vi "nanocal -- nuclear schottky fit V8.vi"() -> ()   [LabVIEW 2021] (continued)
τC\" -> 0.000802475621   ,  \"κ0\" -> 0.000000000773   ,  \"mm1\" -> 0.000163026258   ,  \"mm2\" -> 0.019497997616   ,  \"mm3\" -> 0.165534595934   ,  \"T\" -> 0.190000000000   ,  \"B\" -> 10.000000000000   ,  \"θ\" -> 0.000000000000   ,  \"Reoff\" -> -55142857.142857134400   ,  \"Imoff\" -> 0.000000000000   ,  \"στ1\" -> 0.000058307175   ,  \"στS\" -> 0.000031998048   ,  \"στN\" -> 0.000036682192   ,  \"τ11 \" -> 0.000000000000   ,  \"τ12\" -> 0.000000000000   ,  \"τ22\" -> 0.000000000000   ,  \"τN1\" -> 0.000000000000   ,  \"τN2\" -> 0.000000000000   ,  \"σηlogτ1 \" -> 0.000000000000   ,  \"σηlogτS\" -> 0.000000000000   ,  \"σηlogτN\" -> 0.000000000000   ,  \"σlogτ1\" -> 0.000000000000   ,  \"σlogτS\" -> 0.000000000000   ,  \"σlogτN\" -> 0.000000000000   ,  \"σητ1\" -> 0.000000000000   ,  \"σητS \" -> 0.000000000000   ,  \"σητN\" -> 0.000000000000    |>   , \n\"IDS0424_220526_RAW_cal__sam_\" ->   <|    \"ζ\" -> 0.143096873941   ,  \"τ1\" -> 0.119527741552   ,  \"τS\" -> 0.213771204505   ,  \"τN\" -> 0.133065206622   ,  \"τC\" -> 0.001041786526   ,  \"κ0\" -> 0.000000000890   ,  \"mm1\" -> 0.000129929317   ,  \"mm2\" -> 0.064852834373   ,  \"mm3\" -> 0.452054381716   ,  \"T\" -> 0.190000000000   ,  \"B\" -> 10.000000000000   ,  \"θ\" -> 0.000000000000   ,  \"Reoff\" -> -41461224.489795915800   ,  \"Imoff\" -> 0.000000000000   ,  \"στ1\" -> 0.142328196867   ,  \"στS\" -> 0.153709890516   ,  \"στN\" -> 0.034979737706   ,  \"τ11 \" -> 0.000000000000   ,  \"τ12\" -> 0.000000000000   ,  \"τ22\" -> 0.000000000000   ,  \"τN1\" -> 0.000000000000   ,  \"τN2\" -> 0.000000000000   ,  \"σηlogτ1 \" -> 0.000000000000   ,  \"σηlogτS\" -> 0.000000000000   ,  \"σηlogτN\" -> 0.000000000000   ,  \"σlogτ1\" -> 0.000000000000   ,  \"σlogτS\" -> 0.000000000000   ,  \"σlogτN\" -> 0.000000000000   ,  \"σητ1\" -> 0.000000000000   ,  \"σητS \" -> 0.000000000000   ,  \"σητN\" -> 0.000000000000    |>   , \n\"IDS0425_220526_RAW_cal__ref_\" ->   <|    \"ζ\" -> 0.159335076752   ,  \"τ1\" -> 0.031885685275   ,  \"τS\" -> 0.047996731633   ,  \"τN\" -> 0.019207310502   ,  \"τC\" -> 0.000887935907   ,  \"κ0\" -> 0.000000001118   ,  \"mm1\" -> 0.000120371950   ,  \"mm2\" -> 0.019822778110   ,  \"mm3\" -> 0.090742474469   ,  \"T\" -> 0.250000000000   ,  \"B\" -> 10.000000000000   ,  \"θ\" -> 0.000000000000   ,  \"Reoff\" -> -27579558.011049721400   ,  \"Imoff\" -> 0.000000000000   ,  \"στ1\" -> 0.000105033309   ,  \"στS\" -> 0.000027614157   ,  \"στN\" -> 0.000060474658   ,  \"τ11 \" -> 0.000000000000   ,  \"τ12\" -> 0.000000000000   ,  \"τ22\" -> 0.000000000000   ,  \"τN1\" -> 0.000000000000   ,  \"τN2\" -> 0.000000000000   ,  \"σηlogτ1 \" -> 0.000000000000   ,  \"σηlogτS\" -> 0.000000000000   ,  \"σηlogτN\" -> 0.000000000000   ,  \"σlogτ1\" -> 0.000000000000   ,  \"σlogτS\" -> 0.000000000000   ,  \"σlogτN\" -> 0.000000000000   ,  \"σητ1\" -> 0.000000000000   ,  \"σητS \" -> 0.000000000000   ,  \"σητN\" -> 0.000000000000    |>   , \n\"IDS0425_220526_RAW_cal__sam_\" ->   <|    \"ζ\" -> 0.080613368975   ,  \"τ1\" -> 0.039981630615   ,  \"τS\" -> 0.067451052819   ,  \"τN\" -> 0.024952731947   ,  \"τC\" -> 0.001301901326   ,  \"κ0\" -> 0.000000001270   ,  \"mm1\" -> 0.000095538727   ,  \"mm2\" -> 0.025680137218   ,  \"mm3\" -> 0.115360621158   ,  \"T\" -> 0.250000000000   ,  \"B\" -> 10.000000000000   ,  \"θ\" -> 0.000000000000   ,  \"Reoff\" -> -15077551.020408168400   ,  \"Imoff\" -> 0.000000000000   ,  \"στ1\" -> 0.017921325903   ,  \"στS\" -> 0.008554959302   ,  \"στN\" -> 0.012696106226   ,  \"τ11 \" -> 0.000000000000   ,  \"τ12\" -> 0.000000000000   ,  \"τ22\" -> 0.000000000000   ,  \"τN1\" -> 0.000000000000   ,  \"τN2\" -> 0.000000000000   ,  \"σηlogτ1 \" -> 0.000000000000   ,  \"σηlogτS\" -> 0.000000000000   ,  \"σηlogτN\" -> 0.000000000000   ,  \"σlogτ1\" -> 0.000000000000   ,  \"σlogτS\" -> 0.000000000000   ,  \"σlogτN\" -> 0.000000000000   ,  \"σητ1\" -> 0.000000000000   ,  \"σητS \" -> 0.000000000000   ,  \"σητN\" -> 0.000000000000    |>   , \n\"IDS0426_220526_RAW_cal__ref_\" ->   <|    \"ζ\" -> 0.111460827005   ,  \"τ1\" -> 0.024224453348   ,  \"τS\" -> 0.042028783084   ,  \"τN\" -> 0.009416687783   ,  \"τC\" -> 0.001053496592   ,  \"κ0\" -> 0.000000001428   ,  \"mm1\" -> 0.000103540379   ,  \"mm2\" -> 0.017919606240   ,  \"mm3\" -> 0.064434428916   ,  \"T\" -> 0.300000000000   ,  \"B\" -> 10.000000000000   ,  \"θ\" -> 0.000000000000   ,  \"Reoff\" -> -13408163.265306122600   ,  \"Imoff\" -> 0.000000000000   ,  \"στ1\" -> 0.000203310758   ,  \"στS\" -> 0.000031022481   ,  \"στN\" -> 0.000119793909   ,  \"τ11 \" -> 0.000000000000   ,  \"τ12\" -> 0.000000000000   ,  \"τ22\" -> 0.000000000000   ,  \"τN1\" -> 0.000000000000   ,  \"τN2\" -> 0.000000000000   ,  \"σηlogτ1 \" -> 0.000000000000   ,  \"σηlogτS\" -> 0.000000000000   ,  \"σηlogτN\" -> 0.000000000000   ,  \"σlogτ1\" -> 0.000000000000   ,  \"σlogτS\" -> 0.000000000000   ,  \"σlogτN\" -> 0.000000000000   ,  \"σητ1\" -> 0.000000000000   ,  \"σητS \" -> 0.000000000000   ,  \"σητN\" -> 0.000000000000    |>   , \n\"IDS0426_220526_RAW_cal__sam_\" ->   <|    \"ζ\" -> 0.000000000000   ,  \"τ1\" -> 0.000000000000   ,  \"τS\" -> 0.000000000000   ,  \"τN\" -> 0.000000000000   ,  \"τC\" -> 0.000000000000   ,  \"κ0\" -> 0.000000000000   ,  \"mm1\" -> 0.000000000000   ,  \"mm2\" -> 0.000000000000   ,  \"mm3\" -> 0.000000000000   ,  \"T\" -> 0.300000000000   ,  \"B\" -> 10.000000000000   ,  \"θ\" -> 0.000000000000   ,  \"Reoff\" -> 0.000000000000   ,  \"Imoff\" -> 0.000000000000   ,  \"στ1\" -> 0.000000000000   ,  \"στS\" -> 0.000000000000   ,  \"στN\" -> 0.000000000000   ,  \"τ11 \" -> 0.000000000000   ,  \"τ12\" -> 0.000000000000   ,  \"τ22\" -> 0.000000000000   ,  \"τN1\" -> 0.000000000000   ,  \"τN2\" -> 0.000000000000   ,  \"σηlogτ1 \" -> 0.000000000000   ,  \"σηlogτS\" -> 0.000000000000   ,  \"σηlogτN\" -> 0.000000000000   ,  \"σlogτ1\" -> 0.000000000000   ,  \"σlogτS\" -> 0.000000000000   ,  \"σlogτN\" -> 0.000000000000   ,  \"σητ1\" -> 0.000000000000   ,  \"σητS \" -> 0.000000000000   ,  \"σητN\" -> 0.000000000000    |>   , \n\"IDS0427_220526_RAW_cal__ref_\" ->   <|    \"ζ\" -> 0.410372558234   ,  \"τ1\" -> 0.044042677076   ,  \"τS\" -> 0.102926494068   ,  \"τN\" -> 0.135379226142   ,  \"τC\" -> 0.000829804272   ,  \"κ0\" -> 0.000000000538   ,  \"mm1\" -> 0.000240462729   ,  \"mm2\" -> 0.017682403463   ,  \"mm3\" -> 0.363049463410   ,  \"T\" -> 0.150000000000   ,  \"B\" -> 10.000000000000   ,  \"θ\" -> 0.000000000000   ,  \"Reoff\" -> -106571428.571428567000   ,  \"Imoff\" -> 0.000000000000   ,  \"στ1\" -> 0.000056157157   ,  \"στS\" -> 0.000057678080   ,  \"στN\" -> 0.000041998406   ,  \"τ11 \" -> 0.000000000000   ,  \"τ12\" -> 0.000000000000   ,  \"τ22\" -> 0.000000000000   ,  \"τN1\" -> 0.000000000000   ,  \"τN2\" -> 0.000000000000   ,  \"σηlogτ1 \" -> 0.000000000000   ,  \"σηlogτS\" -> 0.000000000000   ,  \"σηlogτN\" -> 0.000000000000   ,  \"σlogτ1\" -> 0.000000000000   ,  \"σlogτS\" -> 0.000000000000   ,  \"σlogτN\" -> 0.000000000000   ,  \"σητ1\" -> 0.000000000000   ,  \"σητS \" -> 0.000000000000   ,  \"σητN\" -> 0.000000000000    |>   , \n\"IDS0427_220526_RAW_cal__sam_\" ->   <|    \"ζ\" -> 0.000000000000   ,  \"τ1\" -> 0.000000000000   ,  \"τS\" -> 0.000000000000   ,  \"τN\" -> 0.000000000000   ,  \"τC\" -> 0.000000000000   ,  \"κ0\" -> 0.000000000000   ,  \"mm1\" -> 0.000000000000   ,  \"mm2\" -> 0.000000000000   ,  \"mm3\" -> 0.000000000000   ,  \"T\" -> 0.150000000000   ,  \"B\" -> 10.000000000000   ,  \"θ\" -> 0.000000000000   ,  \"Reoff\" -> 0.000000000000   ,  \"Imoff\" -> 0.000000000000   ,  \"στ1\" -> 0.000000000000   ,  \"στS\" -> 0.000000000000   ,  \"στN\" -> 0.000000000000   ,  \"τ11 \" -> 0.000000000000   ,  \"τ12\" -> 0.000000000000   ,  \"τ22\" -> 0.000000000000   ,  \"τN1\" -> 0.000000000000   ,  \"τN2\" -> 0.000000000000   ,  \"σηlogτ1 \" -> 0.000000000000   ,  \"σηlogτS\" -> 0.000000000000   ,  \"σηlogτN\" -> 0.000000000000   ,  \"σlogτ1\" -> 0.000000000000   ,  \"σlogτS\" -> 0.000000000000   ,  \"σlogτN\" -> 0.000000000000   ,  \"σητ1\" -> 0.000000000000   ,  \"σητS \" -> 0.000000000000   ,  \"σητN\" -> 0.000000000000    |>   , \n\"IDS0428_220526_RAW_cal__ref_\" ->   <|    \"ζ\" -> 0.085761087931   ,  \"τ1\" -> 0.025055116447   ,  \"τS\" -> 0.039037181879   ,  \"τN\" -> 0.005587062279   ,  \"τC\" -> 0.001009401057   ,  \"κ0\" -> 0.000000001845   ,  \"mm1\" -> 0.000078014543   ,  \"mm2\" -> 0.019900208864   ,  \"mm3\" -> 0.054537561983   ,  \"T\" -> 0.360000000000   ,  \"B\" -> 10.000000000000   ,  \"θ\" -> 0.000000000000   ,  \"Reoff\" -> -10418232.044198893000   ,  \"Imoff\" -> 0.000000000000   ,  \"στ1\" -> 0.000347384848   ,  \"στS\" -> 0.000031989956   ,  \"στN\" -> 0.000188370043   ,  \"τ11 \" -> 0.000000000000   ,  \"τ12\" -> 0.000000000000   ,  \"τ22\" -> 0.000000000000   ,  \"τN1\" -> 0.000000000000   ,  \"τN2\" -> 0.000000000000   ,  \"σηlogτ1 \" -> 0.000000000000   ,  \"σηlogτS\" -> 0.000000000000   ,  \"σηlogτN\" -> 0.000000000000   ,  \"σlogτ1\" -> 0.000000000000   ,  \"σlogτS\" -> 0.000000000000   ,  \"σlogτN\" -> 0.000000000000   ,  \"σητ1\" -> 0.000000000000   ,  \"σητS \" -> 0.000000000000   ,  \"σητN\" -> 0.000000000000    |>   , \n\"IDS0428_220526_RAW_cal__sam_\" ->   <|    \"ζ\" -> 0.000000000000   ,  \"τ1\" -> 0.000000000000   ,  \"τS\" -> 0.000000000000   ,  \"τN\" -> 0.000000000000   ,  \"τC\" -> 0.000000000000   ,  \"κ0\" -> 0.000000000000   ,  \"mm1\" -> 0.000000000000   ,  \"mm2\" -> 0.000000000000   ,  \"mm3\" -> 0.000000000000   ,  \"T\" -> 0.360000000000   ,  \"B\" -> 10.000000000000   ,  \"θ\" -> 0.000000000000   ,  \"Reoff\" -> 0.000000000000   ,  \"Imoff\" -> 0.000000000000   ,  \"στ1\" -> 0.000000000000   ,  \"στS\" -> 0.000000000000   ,  \"στN\" -> 0.000000000000   ,  \"τ11 \" -> 0.000000000000   ,  \"τ12\" -> 0.000000000000   ,  \"τ22\" -> 0.000000000000   ,  \"τN1\" -> 0.000000000000   ,  \"τN2\" -> 0.000000000000   ,  \"σηlogτ1 \" -> 0.000000000000   ,  \"σηlogτS\" -> 0.000000000000   ,  \"σηlogτN\" -> 0.000000000000   ,  \"σlogτ1\" -> 0.000000000000   ,  \"σlogτS\" -> 0.000000000000   ,  \"σlogτN\" -> 0.000000000000   ,  \"σητ1\" -> 0.000000000000   ,  \"σητS \" -> 0.000000000000   ,  \"σητN\" -> 0.000000000000    |>   , \n\"IDS0429_220526_RAW_cal__ref_\" ->   <|    \"ζ\" -> 0.061793425944   ,  \"τ1\" -> 0.022729976964   ,  \"τS\" -> 0.037992561842   ,  \"τN\" -> 0.003473638845   ,  \"τC\" -> 0.001146343524   ,  \"κ0\" -> 0.000000002261   ,  \"mm1\" -> 0.000064971896   ,  \"mm2\" -> 0.019461604024   ,  \"mm3\" -> 0.048378283857   ,  \"T\" -> 0.420000000000   ,  \"B\" -> 10.000000000000   ,  \"θ\" -> 0.000000000000   ,  \"Reoff\" -> -5435911.602209940560   ,  \"Imoff\" -> 0.000000000000   ,  \"στ1\" -> 0.000628479456   ,  \"στS\" -> 0.000037704094   ,  \"στN\" -> 0.000344539444   ,  \"τ11 \" -> 0.000000000000   ,  \"τ12\" -> 0.000000000000   ,  \"τ22\" -> 0.000000000000   ,  \"τN1\" -> 0.000000000000   ,  \"τN2\" -> 0.000000000000   ,  \"σηlogτ1 \" -> 0.000000000000   ,  \"σηlogτS\" -> 0.000000000000   ,  \"σηlogτN\" -> 0.000000000000   ,  \"σlogτ1\" -> 0.000000000000   ,  \"σlogτS\" -> 0.000000000000   ,  \"σlogτN\" -> 0.000000000000   ,  \"σητ1\" -> 0.000000000000   ,  \"σητS \" -> 0.000000000000   ,  \"σητN\" -> 0.000000000000    |>   , \n\"IDS0429_220526_RAW_cal__sam_\" ->   <|    \"ζ\" -> 0.000000000000   ,  \"τ1\" -> 0.000000000000   ,  \"τS\" -> 0.000000000000   ,  \"τN\" -> 0.000000000000   ,  \"τC\" -> 0.000000000000   ,  \"κ0\" -> 0.000000000000   ,  \"mm1\" -> 0.000000000000   ,  \"mm2\" -> 0.000000000000   ,  \"mm3\" -> 0.000000000000   ,  \"T\" -> 0.420000000000   ,  \"B\" -> 10.000000000000   ,  \"θ\" -> 0.000000000000   ,  \"Reoff\" -> 0.000000000000   ,  \"Imoff\" -> 0.000000000000   ,  \"στ1\" -> 0.000000000000   ,  \"στS\" -> 0.000000000000   ,  \"στN\" -> 0.000000000000   ,  \"τ11 \" -> 0.000000000000   ,  \"τ12\" -> 0.000000000000   ,  \"τ22\" -> 0.000000000000   ,  \"τN1\" -> 0.000000000000   ,  \"τN2\" -> 0.000000000000   ,  \"σηlogτ1 \" -> 0.000000000000   ,  \"σηlogτS\" -> 0.000000000000   ,  \"σηlogτN\" -> 0.000000000000   ,  \"σlogτ1\" -> 0.000000000000   ,  \"σlogτS\" -> 0.000000000000   ,  \"σlogτN\" -> 0.000000000000   ,  \"σητ1\" -> 0.000000000000   ,  \"σητS \" -> 0.000000000000   ,  \"σητN\" -> 0.000000000000    |>   , \n\"IDS0430_220526_RAW_cal__ref_\" ->   <|    \"ζ\" -> 0.045410527771   ,  \"τ1\" -> 0.022224368069   ,  \"τS\" -> 0.038327267568   ,  \"τN\" -> 0.002127889601   ,  \"τC\" -> 0.001500583676   ,  \"κ0\" -> 0.000000002914   ,  \"mm1\" -> 0.000062924210   ,  \"mm2\" -> 0.020129743814   ,  \"mm3\" -> 0.045824530928   ,  \"T\" -> 0.520000000000   ,  \"B\" -> 10.000000000000   ,  \"θ\" -> 0.000000000000   ,  \"Reoff\" -> -3224489.795918375260   ,  \"Imoff\" -> 0.000000000000   ,  \"στ1\" -> 0.001280571461   ,  \"στS\" -> 0.000046989648   ,  \"στN\" -> 0.000705007313   ,  \"τ11 \" -> 0.000000000000   ,  \"τ12\" -> 0.000000000000   ,  \"τ22\" -> 0.000000000000   ,  \"τN1\" -> 0.000000000000   ,  \"τN2\" -> 0.000000000000   ,  \"σηlogτ1 \" -> 0.000000000000   ,  \"σηlogτS\" -> 0.000000000000   ,  \"σηlogτN\" -> 0.000000000000   ,  \"σlogτ1\" -> 0.000000000000   ,  \"σlogτS\" -> 0.000000000000   ,  \"σlogτN\" -> 0.000000000000   ,  \"σητ1\" -> 0.000000000000   ,  \"σητS \" -> 0.000000000000   ,  \"σητN\" -> 0.000000000000    |>   , \n\"IDS0430_220526_RAW_cal__sam_\" ->   <|    \"ζ\" -> 0.000000000000   ,  \"τ1\" -> 0.000000000000   ,  \"τS\" -> 0.000000000000   ,  \"τN\" -> 0.000000000000   ,  \"τC\" -> 0.000000000000   ,  \"κ0\" -> 0.000000000000   ,  \"mm1\" -> 0.000000000000   ,  \"mm2\" -> 0.000000000000   ,  \"mm3\" -> 0.000000000000   ,  \"T\" -> 0.520000000000   ,  \"B\" -> 10.000000000000   ,  \"θ\" -> 0.000000000000   ,  \"Reoff\" -> 0.000000000000   ,  \"Imoff\" -> 0.000000000000   ,  \"στ1\" -> 0.000000000000   ,  \"στS\" -> 0.000000000000   ,  \"στN\" -> 0.000000000000   ,  \"τ11 \" -> 0.000000000000   ,  \"τ12\" -> 0.000000000000   ,  \"τ22\" -> 0.000000000000   ,  \"τN1\" -> 0.000000000000   ,  \"τN2\" -> 0.000000000000   ,  \"σηlogτ1 \" -> 0.000000000000   ,  \"σηlogτS\" -> 0.000000000000   ,  \"σηlogτN\" -> 0.000000000000   ,  \"σlogτ1\" -> 0.000000000000   ,  \"σlogτS\" -> 0.000000000000   ,  \"σlogτN\" -> 0.000000000000   ,  \"σητ1\" -> 0.000000000000   ,  \"σητS \" -> 0.000000000000   ,  \"σητN\" -> 0.000000000000    |>   , \n\"IDS0431_220527_RAW_cal__ref_\" ->   <|    \"ζ\" -> 0.587332924785   ,  \"τ1\" -> 0.048285770693   ,  \"τS\" -> 0.172123299088   ,  \"τN\" -> 0.328986383817   ,  \"τC\" -> 0.000861567300   ,  \"κ0\" -> 0.000000000408   ,  \"mm1\" -> 0.000318149705   ,  \"mm2\" -> 0.015959319465   ,  \"mm3\" -> 0.828297767426   ,  \"T\" -> 0.120000000000   ,  \"B\" -> 10.000000000000   ,  \"θ\" -> 0.000000000000   ,  \"Reoff\" -> -187142857.142857134000   ,  \"Imoff\" -> 0.000000000000   ,  \"στ1\" -> 0.034505118075   ,  \"στS\" -> 0.052461851284   ,  \"στN\" -> 0.093268528407   ,  \"τ11 \" -> 0.000000000000   ,  \"τ12\" -> 0.000000000000   ,  \"τ22\" -> 0.000000000000   ,  \"τN1\" -> 0.000000000000   ,  \"τN2\" -> 0.000000000000   ,  \"σηlogτ1 \" -> 0.000000000000   ,  \"σηlogτS\" -> 0.000000000000   ,  \"σηlogτN\" -> 0.000000000000   ,  \"σlogτ1\" -> 0.000000000000   ,  \"σlogτS\" -> 0.000000000000   ,  \"σlogτN\" -> 0.000000000000   ,  \"σητ1\" -> 0.000000000000   ,  \"σητS \" -> 0.000000000000   ,  \"σητN\" -> 0.000000000000    |>   , \n\"IDS0431_220527_RAW_cal__sam_\" ->   <|    \"ζ\" -> 0.000000000000   ,  \"τ1\" -> 0.000000000000   ,  \"τS\" -> 0.000000000000   ,  \"τN\" -> 0.000000000000   ,  \"τC\" -> 0.000000000000   ,  \"κ0\" -> 0.000000000000   ,  \"mm1\" -> 0.000000000000   ,  \"mm2\" -> 0.000000000000   ,  \"mm3\" -> 0.000000000000   ,  \"T\" -> 0.120000000000   ,  \"B\" -> 10.000000000000   ,  \"θ\" -> 0.000000000000   ,  \"Reoff\" -> 0.000000000000   ,  \"Imoff\" -> 0.000000000000   ,  \"στ1\" -> 0.000000000000   ,  \"στS\" -> 0.000000000000   ,  \"στN\" -> 0.000000000000   ,  \"τ11 \" -> 0.000000000000   ,  \"τ12\" -> 0.000000000000   ,  \"τ22\" -> 0.000000000000   ,  \"τN1\" -> 0.000000000000   ,  \"τN2\" -> 0.000000000000   ,  \"σηlogτ1 \" -> 0.000000000000   ,  \"σηlogτS\" -> 0.000000000000   ,  \"σηlogτN\" -> 0.000000000000   ,  \"σlogτ1\" -> 0.000000000000   ,  \"σlogτS\" -> 0.000000000000   ,  \"σlogτN\" -> 0.000000000000   ,  \"σητ1\" -> 0.000000000000   ,  \"σητS \" -> 0.000000000000   ,  \"σητN\" -> 0.000000000000    |>   , \n\"IDS0432_220527_RAW_cal__ref_\" ->   <|    \"ζ\" -> 0.323198567211   ,  \"τ1\" -> 0.041879804217   ,  \"τS\" -> 0.073059196167   ,  \"τN\" -> 0.074071913735   ,  \"τC\" -> 0.000754510691   ,  \"κ0\" -> 0.000000000676   ,  \"mm1\" -> 0.000183205866   ,  \"mm2\" -> 0.018639437051   ,  \"mm3\" -> 0.218495345806   ,  \"T\" -> 0.170000000000   ,  \"B\" -> 10.000000000000   ,  \"θ\" -> 0.000000000000   ,  \"Reoff\" -> -82571428.571428567200   ,  \"Imoff\" -> 0.000000000000   ,  \"στ1\" -> 0.000050882470   ,  \"στS\" -> 0.000038008306   ,  \"στN\" -> 0.000034915711   ,  \"τ11 \" -> 0.000000000000   ,  \"τ12\" -> 0.000000000000   ,  \"τ22\" -> 0.000000000000   ,  \"τN1\" -> 0.000000000000   ,  \"τN2\" -> 0.000000000000   ,  \"σηlogτ1 \" -> 0.000000000000   ,  \"σηlogτS\" -> 0.000000000000   ,  \"σηlogτN\" -> 0.000000000000   ,  \"σlogτ1\" -> 0.000000000000   ,  \"σlogτS\" -> 0.000000000000   ,  \"σlogτN\" -> 0.000000000000   ,  \"σητ1\" -> 0.000000000000   ,  \"σητS \" -> 0.000000000000   ,  \"σητN\" -> 0.000000000000    |>   , \n\"IDS0432_220527_RAW_cal__sam_\" ->   <|    \"ζ\" -> 0.000000000000   ,  \"τ1\" -> 0.000000000000   ,  \"τS\" -> 0.000000000000   ,  \"τN\" -> 0.000000000000   ,  \"τC\" -> 0.000000000000   ,  \"κ0\" -> 0.000000000000   ,  \"mm1\" -> 0.000000000000   ,  \"mm2\" -> 0.000000000000   ,  \"mm3\" -> 0.000000000000   ,  \"T\" -> 0.170000000000   ,  \"B\" -> 10.000000000000   ,  \"θ\" -> 0.000000000000   ,  \"Reoff\" -> 0.000000000000   ,  \"Imoff\" -> 0.000000000000   ,  \"στ1\" -> 0.000000000000   ,  \"στS\" -> 0.000000000000   ,  \"στN\" -> 0.000000000000   ,  \"τ11 \" -> 0.000000000000   ,  \"τ12\" -> 0.000000000000   ,  \"τ22\" -> 0.000000000000   ,  \"τN1\" -> 0.000000000000   ,  \"τN2\" -> 0.000000000000   ,  \"σηlogτ1 \" -> 0.000000000000   ,  \"σηlogτS\" -> 0.000000000000   ,  \"σηlogτN\" -> 0.000000000000   ,  \"σlogτ1\" -> 0.000000000000   ,  \"σlogτS\" -> 0.000000000000   ,  \"σlogτN\" -> 0.000000000000   ,  \"σητ1\" -> 0.000000000000   ,  \"σητS \" -> 0.000000000000   ,  \"σητN\" -> 0.000000000000    |>   , \n\"IDS0433_220527_RAW_cal__ref_\" ->   <|    \"ζ\" -> 0.036182096392   ,  \"τ1\" -> 0.021229443945   ,  \"τS\" -> 0.040815710128   ,  \"τN\" -> 0.001336208179   ,  \"τC\" -> 0.001738942563   ,  \"κ0\" -> 0.000000003571   ,  \"mm1\" -> 0.000058400724   ,  \"mm2\" -> 0.020067332674   ,  \"mm3\" -> 0.046519716188   ,  \"T\" -> 0.620000000000   ,  \"B\" -> 10.000000000000   ,  \"θ\" -> 0.000000000000   ,  \"Reoff\" -> -1959183.673469394450   ,  \"Imoff\" -> 0.000000000000   ,  \"στ1\" -> 0.002741018217   ,  \"στS\" -> 0.000061676101   ,  \"στN\" -> 0.001584213819   ,  \"τ11 \" -> 0.000000000000   ,  \"τ12\" -> 0.000000000000   ,  \"τ22\" -> 0.000000000000   ,  \"τN1\" -> 0.000000000000   ,  \"τN2\" -> 0.000000000000   ,  \"σηlogτ1 \" -> 0.000000000000   ,  \"σηlogτS\" -> 0.000000000000   ,  \"σηlogτN\" -> 0.000000000000   ,  \"σlogτ1\" -> 0.000000000000   ,  \"σlogτS\" -> 0.000000000000   ,  \"σlogτN\" -> 0.000000000000   ,  \"σητ1\" -> 0.000000000000   ,  \"σητS \" -> 0.000000000000   ,  \"σητN\" -> 0.000000000000    |>   , \n\"IDS0433_220527_RAW_cal__sam_\" ->   <|    \"ζ\" -> 0.000000000000   ,  \"τ1\" -> 0.000000000000   ,  \"τS\" -> 0.000000000000   ,  \"τN\" -> 0.000000000000   ,  \"τC\" -> 0.000000000000   ,  \"κ0\" -> 0.000000000000   ,  \"mm1\" -> 0.000000000000   ,  \"mm2\" -> 0.000000000000   ,  \"mm3\" -> 0.000000000000   ,  \"T\" -> 0.620000000000   ,  \"B\" -> 10.000000000000   ,  \"θ\" -> 0.000000000000   ,  \"Reoff\" -> 0.000000000000   ,  \"Imoff\" -> 0.000000000000   ,  \"στ1\" -> 0.000000000000   ,  \"στS\" -> 0.000000000000   ,  \"στN\" -> 0.000000000000   ,  \"τ11 \" -> 0.000000000000   ,  \"τ12\" -> 0.000000000000   ,  \"τ22\" -> 0.000000000000   ,  \"τN1\" -> 0.000000000000   ,  \"τN2\" -> 0.000000000000   ,  \"σηlogτ1 \" -> 0.000000000000   ,  \"σηlogτS\" -> 0.000000000000   ,  \"σηlogτN\" -> 0.000000000000   ,  \"σlogτ1\" -> 0.000000000000   ,  \"σlogτS\" -> 0.000000000000   ,  \"σlogτN\" -> 0.000000000000   ,  \"σητ1\" -> 0.000000000000   ,  \"σητS \" -> 0.000000000000   ,  \"σητN\" -> 0.000000000000    |>   , \n\"IDS0434_220527_RAW_cal__ref_\" ->   <|    \"ζ\" -> 0.027558689920   ,  \"τ1\" -> 0.020583581485   ,  \"τS\" -> 0.048230388157   ,  \"τN\" -> 0.000508503219   ,  \"τC\" -> 0.001789309584   ,  \"κ0\" -> 0.000000004954   ,  \"mm1\" -> 0.000046358127   ,  \"mm2\" -> 0.020243057541   ,  \"mm3\" -> 0.052165546771   ,  \"T\" -> 0.820000000000   ,  \"B\" -> 10.000000000000   ,  \"θ\" -> 0.000000000000   ,  \"Reoff\" -> -1326530.612244904040   ,  \"Imoff\" -> 0.000000000000   ,  \"στ1\" -> 0.012516710173   ,  \"στS\" -> 0.000096266152   ,  \"στN\" -> 0.007858677235   ,  \"τ11 \" -> 0.000000000000   ,  \"τ12\" -> 0.000000000000   ,  \"τ22\" -> 0.000000000000   ,  \"τN1\" -> 0.000000000000   ,  \"τN2\" -> 0.000000000000   ,  \"σηlogτ1 \" -> 0.000000000000   ,  \"σηlogτS\" -> 0.000000000000   ,  \"σηlogτN\" -> 0.000000000000   ,  \"σlogτ1\" -> 0.000000000000   ,  \"σlogτS\" -> 0.000000000000   ,  \"σlogτN\" -> 0.000000000000   ,  \"σητ1\" -> 0.000000000000   ,  \"σητS \" -> 0.000000000000   ,  \"σητN\" -> 0.000000000000    |>   , \n\"IDS0434_220527_RAW_cal__sam_\" ->   <|    \"ζ\" -> 0.000000000000   ,  \"τ1\" -> 0.000000000000   ,  \"τS\" -> 0.000000000000   ,  \"τN\" -> 0.000000000000   ,  \"τC\" -> 0.000000000000   ,  \"κ0\" -> 0.000000000000   ,  \"mm1\" -> 0.000000000000   ,  \"mm2\" -> 0.000000000000   ,  \"mm3\" -> 0.000000000000   ,  \"T\" -> 0.820000000000   ,  \"B\" -> 10.000000000000   ,  \"θ\" -> 0.000000000000   ,  \"Reoff\" -> 0.000000000000   ,  \"Imoff\" -> 0.000000000000   ,  \"στ1\" -> 0.000000000000   ,  \"στS\" -> 0.000000000000   ,  \"στN\" -> 0.000000000000   ,  \"τ11 \" -> 0.000000000000   ,  \"τ12\" -> 0.000000000000   ,  \"τ22\" -> 0.000000000000   ,  \"τN1\" -> 0.000000000000   ,  \"τN2\" -> 0.000000000000   ,  \"σηlogτ1 \" -> 0.000000000000   ,  \"σηlogτS\" -> 0.000000000000   ,  \"σηlogτN\" -> 0.000000000000   ,  \"σlogτ1\" -> 0.000000000000   ,  \"σlogτS\" -> 0.000000000000   ,  \"σlogτN\" -> 0.000000000000   ,  \"σητ1\" -> 0.000000000000   ,  \"σητS \" -> 0.000000000000   ,  \"σητN\" -> 0.000000000000    |>   , \n\"IDS0435_220527_RAW_cal__ref_\" ->   <|    \"ζ\" -> 0.021047900363   ,  \"τ1\" -> 0.020131753012   ,  \"τS\" -> 0.018766247716   ,  \"τN\" -> 0.000167408006   ,  \"τC\" -> 0.002201803388   ,  \"κ0\" -> 0.000000007032   ,  \"mm1\" -> 0.000040787855   ,  \"mm2\" -> 0.018836680802   ,  \"mm3\" -> 0.022788257164   ,  \"T\" -> 1.120000000000   ,  \"B\" -> 10.000000000000   ,  \"θ\" -> 0.000000000000   ,  \"Reoff\" -> -693877.551020413636   ,  \"Imoff\" -> 0.000000000000   ,  \"στ1\" -> 0.016908966457   ,  \"στS\" -> 0.000075633195   ,  \"στN\" -> 0.007369905753   ,  \"τ11 \" -> 0.000000000000   ,  \"τ12\" -> 0.000000000000   ,  \"τ22\" -> 0.000000000000   ,  \"τN1\" -> 0.000000000000   ,  \"τN2\" -> 0.000000000000   ,  \"σηlogτ1 \" -> 0.000000000000   ,  \"σηlogτS\" -> 0.000000000000   ,  \"σηlogτN\" -> 0.000000000000   ,  \"σlogτ1\" -> 0.000000000000   ,  \"σlogτS\" -> 0.000000000000   ,  \"σlogτN\" -> 0.000000000000   ,  \"σητ1\" -> 0.000000000000   ,  \"σητS \" -> 0.000000000000   ,  \"σητN\" -> 0.000000000000    |>   , \n\"IDS0435_220527_RAW_cal__sam_\" ->   <|    \"ζ\" -> 0.000000000000   ,  \"τ1\" -> 0.000000000000   ,  \"τS\" -> 0.000000000000   ,  \"τN\" -> 0.000000000000   ,  \"τC\" -> 0.000000000000   ,  \"κ0\" -> 0.000000000000   ,  \"mm1\" -> 0.000000000000   ,  \"mm2\" -> 0.000000000000   ,  \"mm3\" -> 0.000000000000   ,  \"T\" -> 1.120000000000   ,  \"B\" -> 10.000000000000   ,  \"θ\" -> 0.000000000000   ,  \"Reoff\" -> 0.000000000000   ,  \"Imoff\" -> 0.000000000000   ,  \"στ1\" -> 0.000000000000   ,  \"στS\" -> 0.000000000000   ,  \"στN\" -> 0.000000000000   ,  \"τ11 \" -> 0.000000000000   ,  \"τ12\" -> 0.000000000000   ,  \"τ22\" -> 0.000000000000   ,  \"τN1\" -> 0.000000000000   ,  \"τN2\" -> 0.000000000000   ,  \"σηlogτ1 \" -> 0.000000000000   ,  \"σηlogτS\" -> 0.000000000000   ,  \"σηlogτN\" -> 0.000000000000   ,  \"σlogτ1\" -> 0.000000000000   ,  \"σlogτS\" -> 0.000000000000   ,  \"σlogτN\" -> 0.000000000000   ,  \"σητ1\" -> 0.000000000000   ,  \"σητS \" -> 0.000000000000   ,  \"σητN\" -> 0.000000000000    |>   , \n\"IDS0436_220527_RAW_cal__ref_\" ->   <|    \"ζ\" -> 0.021136828909   ,  \"τ1\" -> 0.020409850300   ,  \"τS\" -> 0.013072920325   ,  \"τN\" -> 0.000033999187   ,  \"τC\" -> 0.001843360192   ,  \"κ0\" -> 0.000000012245   ,  \"mm1\" -> 0.000033600976   ,  \"mm2\" -> 0.015061266105   ,  \"mm3\" -> 0.020542301639   ,  \"T\" -> 1.900000000000   ,  \"B\" -> 10.000000000000   ,  \"θ\" -> 0.000000000000   ,  \"Reoff\" -> -693877.551020413636   ,  \"Imoff\" -> 0.000000000000   ,  \"στ1\" -> 0.104903022398   ,  \"στS\" -> 0.000108844468   ,  \"στN\" -> 0.048413381920   ,  \"τ11 \" -> 0.000000000000   ,  \"τ12\" -> 0.000000000000   ,  \"τ22\" -> 0.000000000000   ,  \"τN1\" -> 0.000000000000   ,  \"τN2\" -> 0.000000000000   ,  \"σηlogτ1 \" -> 0.000000000000   ,  \"σηlogτS\" -> 0.000000000000   ,  \"σηlogτN\" -> 0.000000000000   ,  \"σlogτ1\" -> 0.000000000000   ,  \"σlogτS\" -> 0.000000000000   ,  \"σlogτN\" -> 0.000000000000   ,  \"σητ1\" -> 0.000000000000   ,  \"σητS \" -> 0.000000000000   ,  \"σητN\" -> 0.000000000000    |>   , \n\"IDS0436_220527_RAW_cal__sam_\" ->   <|    \"ζ\" -> 0.000000000000   ,  \"τ1\" -> 0.000000000000   ,  \"τS\" -> 0.000000000000   ,  \"τN\" -> 0.000000000000   ,  \"τC\" -> 0.000000000000   ,  \"κ0\" -> 0.000000000000   ,  \"mm1\" -> 0.000000000000   ,  \"mm2\" -> 0.000000000000   ,  \"mm3\" -> 0.000000000000   ,  \"T\" -> 1.900000000000   ,  \"B\" -> 10.000000000000   ,  \"θ\" -> 0.000000000000   ,  \"Reoff\" -> 0.000000000000   ,  \"Imoff\" -> 0.000000000000   ,  \"στ1\" -> 0.000000000000   ,  \"στS\" -> 0.000000000000   ,  \"στN\" -> 0.000000000000   ,  \"τ11 \" -> 0.000000000000   ,  \"τ12\" -> 0.000000000000   ,  \"τ22\" -> 0.000000000000   ,  \"τN1\" -> 0.000000000000   ,  \"τN2\" -> 0.000000000000   ,  \"σηlogτ1 \" -> 0.000000000000   ,  \"σηlogτS\" -> 0.000000000000   ,  \"σηlogτN\" -> 0.000000000000   ,  \"σlogτ1\" -> 0.000000000000   ,  \"σlogτS\" -> 0.000000000000   ,  \"σlogτN\" -> 0.000000000000   ,  \"σητ1\" -> 0.000000000000   ,  \"σητS \" -> 0.000000000000   ,  \"σητN\" -> 0.000000000000    |>   , \n\"IDS0437_220527_RAW_cal__ref_\" ->   <|    \"ζ\" -> 0.018218676820   ,  \"τ1\" -> 0.021192441763   ,  \"τS\" -> 0.009662387372   ,  \"τN\" -> 0.000008791358   ,  \"τC\" -> 0.001686673975   ,  \"κ0\" -> 0.000000021992   ,  \"mm1\" -> 0.000025820332   ,  \"mm2\" -> 0.011488682872   ,  \"mm3\" -> 0.021211987344   ,  \"T\" -> 3.100000000000   ,  \"B\" -> 10.000000000000   ,  \"θ\" -> 0.000000000000   ,  \"Reoff\" -> -326530.612244898453   ,  \"Imoff\" -> 0.000000000000   ,  \"στ1\" -> 0.606338266811   ,  \"στS\" -> 0.000173040998   ,  \"στN\" -> 0.325575671628   ,  \"τ11 \" -> 0.000000000000   ,  \"τ12\" -> 0.000000000000   ,  \"τ22\" -> 0.000000000000   ,  \"τN1\" -> 0.000000000000   ,  \"τN2\" -> 0.000000000000   ,  \"σηlogτ1 \" -> 0.000000000000   ,  \"σηlogτS\" -> 0.000000000000   ,  \"σηlogτN\" -> 0.000000000000   ,  \"σlogτ1\" -> 0.000000000000   ,  \"σlogτS\" -> 0.000000000000   ,  \"σlogτN\" -> 0.000000000000   ,  \"σητ1\" -> 0.000000000000   ,  \"σητS \" -> 0.000000000000   ,  \"σητN\" -> 0.000000000000    |>   , \n\"IDS0437_220527_RAW_cal__sam_\" ->   <|    \"ζ\" -> 0.000000000000   ,  \"τ1\" -> 0.000000000000   ,  \"τS\" -> 0.000000000000   ,  \"τN\" -> 0.000000000000   ,  \"τC\" -> 0.000000000000   ,  \"κ0\" -> 0.000000000000   ,  \"mm1\" -> 0.000000000000   ,  \"mm2\" -> 0.000000000000   ,  \"mm3\" -> 0.000000000000   ,  \"T\" -> 3.100000000000   ,  \"B\" -> 10.000000000000   ,  \"θ\" -> 0.000000000000   ,  \"Reoff\" -> 0.000000000000   ,  \"Imoff\" -> 0.000000000000   ,  \"στ1\" -> 0.000000000000   ,  \"στS\" -> 0.000000000000   ,  \"στN\" -> 0.000000000000   ,  \"τ11 \" -> 0.000000000000   ,  \"τ12\" -> 0.000000000000   ,  \"τ22\" -> 0.000000000000   ,  \"τN1\" -> 0.000000000000   ,  \"τN2\" -> 0.000000000000   ,  \"σηlogτ1 \" -> 0.000000000000   ,  \"σηlogτS\" -> 0.000000000000   ,  \"σηlogτN\" -> 0.000000000000   ,  \"σlogτ1\" -> 0.000000000000   ,  \"σlogτS\" -> 0.000000000000   ,  \"σlogτN\" -> 0.000000000000   ,  \"σητ1\" -> 0.000000000000   ,  \"σητS \" -> 0.000000000000   ,  \"σητN\" -> 0.000000000000    |>   , \n\"IDS0438_220527_RAW_cal__ref_\" ->   <|    \"ζ\" -> 0.017431684106   ,  \"τ1\" -> 0.021485980533   ,  \"τS\" -> 0.006444404712   ,  \"τN\" -> 0.000001115072   ,  \"τC\" -> 0.001296544694   ,  \"κ0\" -> 0.000000054868   ,  \"mm1\" -> 0.000018590347   ,  \"mm2\" -> 0.007834045159   ,  \"mm3\" -> 0.021487765770   ,  \"T\" -> 5.700000000000   ,  \"B\" -> 10.000000000000   ,  \"θ\" -> 0.000000000000   ,  \"Reoff\" -> -102040.816326530650   ,  \"Imoff\" -> 0.000000000000   ,  \"στ1\" -> 10.046797203263   ,  \"στS\" -> 0.000382400636   ,  \"στN\" -> 6.574038852871   ,  \"τ11 \" -> 0.000000000000   ,  \"τ12\" -> 0.000000000000   ,  \"τ22\" -> 0.000000000000   ,  \"τN1\" -> 0.000000000000   ,  \"τN2\" -> 0.000000000000   ,  \"σηlogτ1 \" -> 0.000000000000   ,  \"σηlogτS\" -> 0.000000000000   ,  \"σηlogτN\" -> 0.000000000000   ,  \"σlogτ1\" -> 0.000000000000   ,  \"σlogτS\" -> 0.000000000000   ,  \"σlogτN\" -> 0.000000000000   ,  \"σητ1\" -> 0.000000000000   ,  \"σητS \" -> 0.000000000000   ,  \"σητN\" -> 0.000000000000    |>   , \n\"IDS0438_220527_RAW_cal__sam_\" ->   <|    \"ζ\" -> 0.000000000000   ,  \"τ1\" -> 0.000000000000   ,  \"τS\" -> 0.000000000000   ,  \"τN\" -> 0.000000000000   ,  \"τC\" -> 0.000000000000   ,  \"κ0\" -> 0.000000000000   ,  \"mm1\" -> 0.000000000000   ,  \"mm2\" -> 0.000000000000   ,  \"mm3\" -> 0.000000000000   ,  \"T\" -> 5.700000000000   ,  \"B\" -> 10.000000000000   ,  \"θ\" -> 0.000000000000   ,  \"Reoff\" -> 0.000000000000   ,  \"Imoff\" -> 0.000000000000   ,  \"στ1\" -> 0.000000000000   ,  \"στS\" -> 0.000000000000   ,  \"στN\" -> 0.000000000000   ,  \"τ11 \" -> 0.000000000000   ,  \"τ12\" -> 0.000000000000   ,  \"τ22\" -> 0.000000000000   ,  \"τN1\" -> 0.000000000000   ,  \"τN2\" -> 0.000000000000   ,  \"σηlogτ1 \" -> 0.000000000000   ,  \"σηlogτS\" -> 0.000000000000   ,  \"σηlogτN\" -> 0.000000000000   ,  \"σlogτ1\" -> 0.000000000000   ,  \"σlogτS\" -> 0.000000000000   ,  \"σlogτN\" -> 0.000000000000   ,  \"σητ1\" -> 0.000000000000   ,  \"σητS \" -> 0.000000000000   ,  \"σητN\" -> 0.000000000000    |>   , \n\"IDS0439_220527_RAW_cal__ref_\" ->   <|    \"ζ\" -> 0.020689762158   ,  \"τ1\" -> 0.020173245371   ,  \"τS\" -> 0.016460366975   ,  \"τN\" -> 0.000108383965   ,  \"τC\" -> 0.002269516134   ,  \"κ0\" -> 0.000000008014   ,  \"mm1\" -> 0.000040615587   ,  \"mm2\" -> 0.018076419780   ,  \"mm3\" -> 0.021237280594   ,  \"T\" -> 1.280000000000   ,  \"B\" -> 10.000000000000   ,  \"θ\" -> 0.000000000000   ,  \"Reoff\" -> -693877.551020413636   ,  \"Imoff\" -> 0.000000000000   ,  \"στ1\" -> 0.026382279161   ,  \"στS\" -> 0.000081346280   ,  \"στN\" -> 0.011459824144   ,  \"τ11 \" -> 0.000000000000   ,  \"τ12\" -> 0.000000000000   ,  \"τ22\" -> 0.000000000000   ,  \"τN1\" -> 0.000000000000   ,  \"τN2\" -> 0.000000000000   ,  \"σηlogτ1 \" -> 0.000000000000   ,  \"σηlogτS\" -> 0.000000000000   ,  \"σηlogτN\" -> 0.000000000000   ,  \"σlogτ1\" -> 0.000000000000   ,  \"σlogτS\" -> 0.000000000000   ,  \"σlogτN\" -> 0.000000000000   ,  \"σητ1\" -> 0.000000000000   ,  \"σητS \" -> 0.000000000000   ,  \"σητN\" -> 0.000000000000    |>   , \n\"IDS0439_220527_RAW_cal__sam_\" ->   <|    \"ζ\" -> 0.000000000000   ,  \"τ1\" -> 0.000000000000   ,  \"τS\" -> 0.000000000000   ,  \"τN\" -> 0.000000000000   ,  \"τC\" -> 0.000000000000   ,  \"κ0\" -> 0.000000000000   ,  \"mm1\" -> 0.000000000000   ,  \"mm2\" -> 0.000000000000   ,  \"mm3\" -> 0.000000000000   ,  \"T\" -> 1.280000000000   ,  \"B\" -> 10.000000000000   ,  \"θ\" -> 0.000000000000   ,  \"Reoff\" -> 0.000000000000   ,  \"Imoff\" -> 0.000000000000   ,  \"στ1\" -> 0.000000000000   ,  \"στS\" -> 0.000000000000   ,  \"στN\" -> 0.000000000000   ,  \"τ11 \" -> 0.000000000000   ,  \"τ12\" -> 0.000000000000   ,  \"τ22\" -> 0.000000000000   ,  \"τN1\" -> 0.000000000000   ,  \"τN2\" -> 0.000000000000   ,  \"σηlogτ1 \" -> 0.000000000000   ,  \"σηlogτS\" -> 0.000000000000   ,  \"σηlogτN\" -> 0.000000000000   ,  \"σlogτ1\" -> 0.000000000000   ,  \"σlogτS\" -> 0.000000000000   ,  \"σlogτN\" -> 0.000000000000   ,  \"σητ1\" -> 0.000000000000   ,  \"σητS \" -> 0.000000000000   ,  \"σητN\" -> 0.000000000000    |>   , \n\"IDS0441_220527_RAW_cal__ref_\" ->   <|    \"ζ\" -> 0.259547281535   ,  \"τ1\" -> 0.090051958838   ,  \"τS\" -> 0.023394515499   ,  \"τN\" -> 0.011063320933   ,  \"τC\" -> 0.000755636081   ,  \"κ0\" -> 0.000000000806   ,  \"mm1\" -> 0.000152584106   ,  \"mm2\" -> 0.024779990454   ,  \"mm3\" -> 0.109276294565   ,  \"T\" -> 0.200000000000   ,  \"B\" -> 6.000000000000   ,  \"θ\" -> 0.000000000000   ,  \"Reoff\" -> -55142857.142857134400   ,  \"Imoff\" -> 0.000000000000   ,  \"στ1\" -> 0.000065846080   ,  \"στS\" -> 0.000007078424   ,  \"στN\" -> 0.000042629907   ,  \"τ11 \" -> 0.000000000000   ,  \"τ12\" -> 0.000000000000   ,  \"τ22\" -> 0.000000000000   ,  \"τN1\" -> 0.000000000000   ,  \"τN2\" -> 0.000000000000   ,  \"σηlogτ1 \" -> 0.000000000000   ,  \"σηlogτS\" -> 0.000000000000   ,  \"σηlogτN\" -> 0.000000000000   ,  \"σlogτ1\" -> 0.000000000000   ,  \"σlogτS\" -> 0.000000000000   ,  \"σlogτN\" -> 0.000000000000   ,  \"σητ1\" -> 0.000000000000   ,  \"σητS \" -> 0.000000000000   ,  \"σητN\" -> 0.000000000000    |>   , \n\"IDS0441_220527_RAW_cal__sam_\" ->   <|    \"ζ\" -> 0.000000000000   ,  \"τ1\" -> 0.000000000000   ,  \"τS\" -> 0.000000000000   ,  \"τN\" -> 0.000000000000   ,  \"τC\" -> 0.000000000000   ,  \"κ0\" -> 0.000000000000   ,  \"mm1\" -> 0.000000000000   ,  \"mm2\" -> 0.000000000000   ,  \"mm3\" -> 0.000000000000   ,  \"T\" -> 0.200000000000   ,  \"B\" -> 6.000000000000   ,  \"θ\" -> 0.000000000000   ,  \"Reoff\" -> 0.000000000000   ,  \"Imoff\" -> 0.000000000000   ,  \"στ1\" -> 0.000000000000   ,  \"στS\" -> 0.000000000000   ,  \"στN\" -> 0.000000000000   ,  \"τ11 \" -> 0.000000000000   ,  \"τ12\" -> 0.000000000000   ,  \"τ22\" -> 0.000000000000   ,  \"τN1\" -> 0.000000000000   ,  \"τN2\" -> 0.000000000000   ,  \"σηlogτ1 \" -> 0.000000000000   ,  \"σηlogτS\" -> 0.000000000000   ,  \"σηlogτN\" -> 0.000000000000   ,  \"σlogτ1\" -> 0.000000000000   ,  \"σlogτS\" -> 0.000000000000   ,  \"σlogτN\" -> 0.000000000000   ,  \"σητ1\" -> 0.000000000000   ,  \"σητS \" -> 0.000000000000   ,  \"σητN\" -> 0.000000000000    |>   , \n\"IDS0442_220528_RAW_cal__ref_\" ->   <|    \"ζ\" -> 0.735384150103   ,  \"τ1\" -> 0.108338779465   ,  \"τS\" -> 0.047519369328   ,  \"τN\" -> 0.067177831224   ,  \"τC\" -> 0.000775501917   ,  \"κ0\" -> 0.000000000463   ,  \"mm1\" -> 0.000326839822   ,  \"mm2\" -> 0.032642743748   ,  \"mm3\" -> 0.275188401711   ,  \"T\" -> 0.120000000000   ,  \"B\" -> 6.000000000000   ,  \"θ\" -> 0.000000000000   ,  \"Reoff\" -> -187755102.040816367000   ,  \"Imoff\" -> 0.000000000000   ,  \"στ1\" -> 0.000025892461   ,  \"στS\" -> 0.000015077221   ,  \"στN\" -> 0.000012991110   ,  \"τ11 \" -> 0.000000000000   ,  \"τ12\" -> 0.000000000000   ,  \"τ22\" -> 0.000000000000   ,  \"τN1\" -> 0.000000000000   ,  \"τN2\" -> 0.000000000000   ,  \"σηlogτ1 \" -> 0.000000000000   ,  \"σηlogτS\" -> 0.000000000000   ,  \"σηlogτN\" -> 0.000000000000   ,  \"σlogτ1\" -> 0.000000000000   ,  \"σlogτS\" -> 0.000000000000   ,  \"σlogτN\" -> 0.000000000000   ,  \"σητ1\" -> 0.000000000000   ,  \"σητS \" -> 0.000000000000   ,  \"σητN\" -> 0.000000000000    |>   , \n\"IDS0442_220528_RAW_cal__sam_\" ->   <|    \"ζ\" -> 0.000000000000   ,  \"τ1\" -> 0.000000000000   ,  \"τS\" -> 0.000000000000   ,  \"τN\" -> 0.000000000000   ,  \"τC\" -> 0.000000000000   ,  \"κ0\" -> 0.000000000000   ,  \"mm1\" -> 0.000000000000   ,  \"mm2\" -> 0.000000000000   ,  \"mm3\" -> 0.000000000000   ,  \"T\" -> 0.120000000000   ,  \"B\" -> 6.000000000000   ,  \"θ\" -> 0.000000000000   ,  \"Reoff\" -> 0.000000000000   ,  \"Imoff\" -> 0.000000000000   ,  \"στ1\" -> 0.000000000000   ,  \"στS\" -> 0.000000000000   ,  \"στN\" -> 0.000000000000   ,  \"τ11 \" -> 0.000000000000   ,  \"τ12\" -> 0.000000000000   ,  \"τ22\" -> 0.000000000000   ,  \"τN1\" -> 0.000000000000   ,  \"τN2\" -> 0.000000000000   ,  \"σηlogτ1 \" -> 0.000000000000   ,  \"σηlogτS\" -> 0.000000000000   ,  \"σηlogτN\" -> 0.000000000000   ,  \"σlogτ1\" -> 0.000000000000   ,  \"σlogτS\" -> 0.000000000000   ,  \"σlogτN\" -> 0.000000000000   ,  \"σητ1\" -> 0.000000000000   ,  \"σητS \" -> 0.000000000000   ,  \"σητN\" -> 0.000000000000    |>   , \n\"IDS0443_220528_RAW_cal__ref_\" ->   <|    \"ζ\" -> 0.466849978286   ,  \"τ1\" -> 0.114460003780   ,  \"τS\" -> 0.033572722745   ,  \"τN\" -> 0.036649272390   ,  \"τC\" -> 0.000752381587   ,  \"κ0\" -> 0.000000000618   ,  \"mm1\" -> 0.000236972471   ,  \"mm2\" -> 0.030357978789   ,  \"mm3\" -> 0.187622566146   ,  \"T\" -> 0.150000000000   ,  \"B\" -> 6.000000000000   ,  \"θ\" -> 0.000000000000   ,  \"Reoff\" -> -104489795.918367386000   ,  \"Imoff\" -> 0.000000000000   ,  \"στ1\" -> 0.000032948033   ,  \"στS\" -> 0.000009842320   ,  \"στN\" -> 0.000019499617   ,  \"τ11 \" -> 0.000000000000   ,  \"τ12\" -> 0.000000000000   ,  \"τ22\" -> 0.000000000000   ,  \"τN1\" -> 0.000000000000   ,  \"τN2\" -> 0.000000000000   ,  \"σηlogτ1 \" -> 0.000000000000   ,  \"σηlogτS\" -> 0.000000000000   ,  \"σηlogτN\" -> 0.000000000000   ,  \"σlogτ1\" -> 0.000000000000   ,  \"σlogτS\" -> 0.000000000000   ,  \"σlogτN\" -> 0.000000000000   ,  \"σητ1\" -> 0.000000000000   ,  \"σητS \" -> 0.000000000000   ,  \"σητN\" -> 0.000000000000    |>   , \n\"IDS0443_220528_RAW_cal__sam_\" ->   <|    \"ζ\" -> 0.000000000000   ,  \"τ1\" -> 0.000000000000   ,  \"τS\" -> 0.000000000000   ,  \"τN\" -> 0.000000000000   ,  \"τC\" -> 0.000000000000   ,  \"κ0\" -> 0.000000000000   ,  \"mm1\" -> 0.000000000000   ,  \"mm2\" -> 0.000000000000   ,  \"mm3\" -> 0.000000000000   ,  \"T\" -> 0.150000000000   ,  \"B\" -> 6.000000000000   ,  \"θ\" -> 0.000000000000   ,  \"Reoff\" -> 0.000000000000   ,  \"Imoff\" -> 0.000000000000   ,  \"στ1\" -> 0.000000000000   ,  \"στS\" -> 0.000000000000   ,  \"στN\" -> 0.000000000000   ,  \"τ11 \" -> 0.000000000000   ,  \"τ12\" -> 0.000000000000   ,  \"τ22\" -> 0.000000000000   ,  \"τN1\" -> 0.000000000000   ,  \"τN2\" -> 0.000000000000   ,  \"σηlogτ1 \" -> 0.000000000000   ,  \"σηlogτS\" -> 0.000000000000   ,  \"σηlogτN\" -> 0.000000000000   ,  \"σlogτ1\" -> 0.000000000000   ,  \"σlogτS\" -> 0.000000000000   ,  \"σlogτN\" -> 0.000000000000   ,  \"σητ1\" -> 0.000000000000   ,  \"σητS \" -> 0.000000000000   ,  \"σητN\" -> 0.000000000000    |>   , \n\"IDS0444_220528_RAW_cal__ref_\" ->   <|    \"ζ\" -> 0.358662546847   ,  \"τ1\" -> 0.106553219488   ,  \"τS\" -> 0.027408143285   ,  \"τN\" -> 0.021718202287   ,  \"τC\" -> 0.000737226572   ,  \"κ0\" -> 0.000000000747   ,  \"mm1\" -> 0.000191801290   ,  \"mm2\" -> 0.027513397927   ,  \"mm3\" -> 0.146331372634   ,  \"T\" -> 0.170000000000   ,  \"B\" -> 6.000000000000   ,  \"θ\" -> 0.000000000000   ,  \"Reoff\" -> -71183673.469387769700   ,  \"Imoff\" -> 0.000000000000   ,  \"στ1\" -> 0.000046007693   ,  \"στS\" -> 0.000008627016   ,  \"στN\" -> 0.000029243176   ,  \"τ11 \" -> 0.000000000000   ,  \"τ12\" -> 0.000000000000   ,  \"τ22\" -> 0.000000000000   ,  \"τN1\" -> 0.000000000000   ,  \"τN2\" -> 0.000000000000   ,  \"σηlogτ1 \" -> 0.000000000000   ,  \"σηlogτS\" -> 0.000000000000   ,  \"σηlogτN\" -> 0.000000000000   ,  \"
